vi "Global 1.vi"() -> ()   [LabVIEW 2015]
uses:
  <vilib>/Analysis/Matrix/Datatypes/RealMatrix.ctl
  <vilib>/Analysis/Matrix/NI_Matrix.lvlib
panel:
  out "LCM_CAN_EYE_RAW_T":T1={"hash"=-386282380061490012, "sys time"=0, "mobileye time"=0, "ID"=0, "data"=[]} {"hash" format="%016x"}
  out "Door":bool
  out "Right light":bool
  out "Left light":bool
  out "time":u32
  out "WHL_SPD_FL":dbl
  out "WHL_SPD_FR":dbl
  out "WHL_SPD_RL":dbl
  out "WHL_SPD_RR":dbl
  out "LCM PC":T2={"connection ID"=refnum, "net address"=0, "port"=7667}
  out "CON_INPUT_T":T3={"hash"=7122929053877479277, "sys time"=0, "ref_vel"=0.0, "ref_steer"=0.0} {"hash" format="%016x"}
  out "LCM_CON_T":T4={"hash"=4999688090526594712, "sys time"=0, "Auto"=FALSE, "Run"=FALSE, "Solenoid"=FALSE, "T lim"=FALSE, "brk_enc"=0, "B PWM"=0, "T PWM"=0, "ref_vel"=0.0, "ref_bkr_enc"=0.0, "ref_apv"=0.0, "ref_steer"=0.0} {"hash" format="%016x"}
  out "LCM_EYE_RAW_T":T5={"hash"=-8920902524919788889, "sys time"=0, "mobileye"=[]} {"hash" format="%016x"}
  out "LCM_POS_T":T6={"hash"=8611666821338907869, "sys time"=0, "dt"=0.0, "x"=0.0, "y"=0.0, "speed"=0.0, "heading"=0.0, "yaw_rate"=0.0} {"hash" format="%016x"}
  out "LCM_CAN_T":T7={"hash"=4925705798588944810, "sys time"=0, "time"=0.0, "yaw_rate"=0.0, "mdps torque"=0.0, "mdps str_ang"=0.0, "VS_CAN"=0.0, "lat_accel"=0.0, "mcp"=0.0, "accel pedal value"=0.0, "tps"=0.0, "odometer"=0.0, "battery voltage"=0.0, "WHL_SPD_RR"=0.0, "WHL_SPD_RL"=0.0, "WHL_SPD_FR"=0.0, "WHL_SPD_FL"=0.0} {"hash" format="%016x"}
  out "LCM":T2={"connection ID"=refnum, "net address"=0, "port"=7667}
  out "LCM_GGA_T":T8={"hash"=1114363806672425932, "sys time"=0, "time"=0.0, "x"=0.0, "y"=0.0, "h"=0.0, "numSV"=0, "postype"=0, "lag"=0, "hordev"=0.0, "lat"=0.0, "lon"=0.0, "hgt"=0.0, "map_idx"=0} {"hash" format="%016x"}
  out "LCM_RMC_T":T9={"hash"=2469426948741950939, "sys time"=0, "time"=0.0, "speed"=0.0, "heading"=0.0, "lat"=0.0, "lon"=0.0} {"hash" format="%016x"}
  out "K":T10=[[1.0, 0.0, 0.0], [0.0, 1.0, 0.0], [0.0, 0.0, 0.05], [0.0, 0.0, 0.0], [0.0, 0.0, 0.0]]
  out "Pp":T10=[[1.0, 0.0, 0.0, 0.0, 0.0], [0.0, 1.0, 0.0, 0.0, 0.0], [0.0, 0.0, 0.05, 0.0, 0.0], [0.0, 0.0, 0.0, 0.0188, 0.0], [0.0, 0.0, 0.0, 0.0, 0.0017]]
  out "H":T10=[[1.0, 0.0, 0.0, 0.0, 0.0], [0.0, 1.0, 0.0, 0.0, 0.0], [0.0, 0.0, 0.0, 1.0, 0.0]]
  out "R":T10=[[10.0, 0.0, 0.0], [0.0, 10.0, 0.0], [0.0, 0.0, 0.5]]
  out "Q":T10=[[0.5, 0.0, 0.0, 0.0, 0.0], [0.0, 0.5, 0.0, 0.0, 0.0], [0.0, 0.0, 0.1, 0.0, 0.0], [0.0, 0.0, 0.0, 0.0341, 0.0], [0.0, 0.0, 0.0, 0.0, 0.0017]]
  out "P":T10=[[1.0, 0.0, 0.0, 0.0, 0.0], [0.0, 1.0, 0.0, 0.0, 0.0], [0.0, 0.0, 0.1, 0.0, 0.0], [0.0, 0.0, 0.0, 0.0341, 0.0], [0.0, 0.0, 0.0, 0.0, 0.0017]]
  out "gps_pos 2":dbl[](array[numeric]) format="%#_19f"
  out "gps_vel 2":dbl[](array[numeric]) format="%#_19f"
  out "gps_pos 1":dbl[](array[numeric]) format="%#_19f"
  out "gps_vel 1":dbl[](array[numeric]) format="%#_19f"
  out "ts":dbl
  out "mcp":u16
  out "Ref Brk FULL":dbl=80.0
  out "Ref Brk Enc":dbl
  out "Ref APS":dbl
  out "VS_CAN":dbl
  out "Brake Encoder mcp":dbl
  out "mdps str_ang":dbl
  out "mdps torque":dbl
  out "vs_esc":dbl
  out "odometer":dbl
  out "gear selector disp":u8
  out "battery voltage":dbl
  out "brake_act_can":bool
  out "accel pedal value":dbl
  out "tps":dbl
  out "lat_accel":dbl
  out "yaw_rate":dbl
  out "Auto":bool
  out "Run":bool
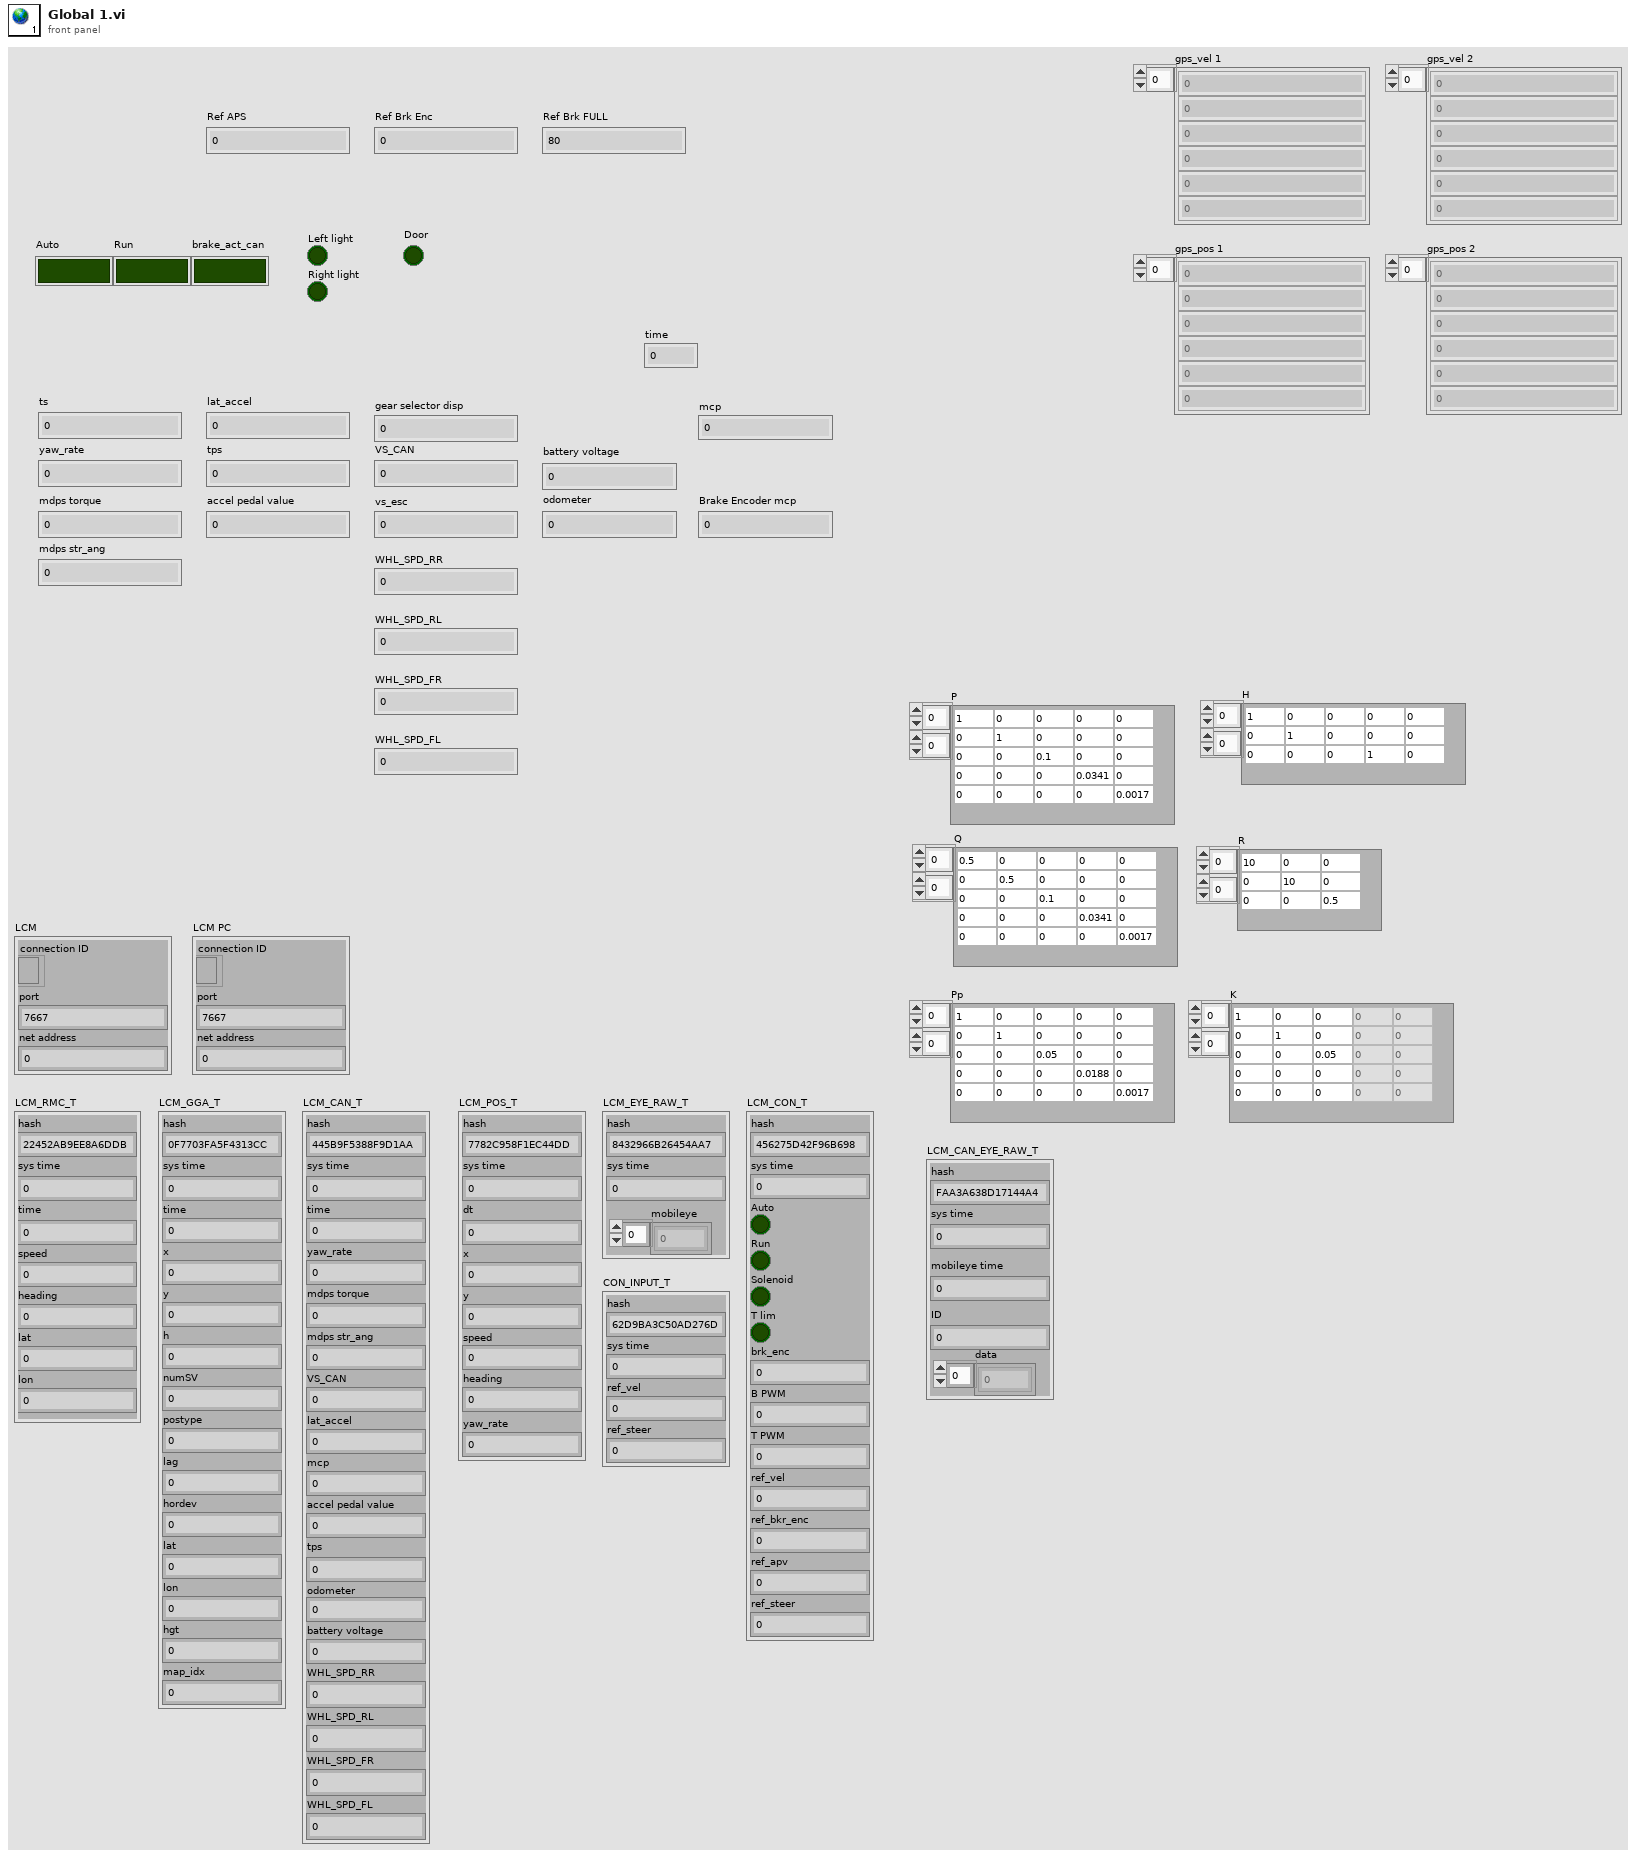
[diagram p1: front panel]
types:
  T1 = cluster{"hash":i64, "sys time":i64, "mobileye time":u32, "ID":u32, "data":u8[]}
  T2 = cluster{"connection ID":refnum<k16>, "net address":u32, "port":u16}
  T3 = cluster{"hash":i64, "sys time":i64, "ref_vel":dbl, "ref_steer":dbl}
  T4 = cluster{"hash":i64, "sys time":i64, "Auto":bool, "Run":bool, "Solenoid":bool, "T lim":bool, "brk_enc":u8, "B PWM":u16, "T PWM":u16, "ref_vel":dbl, "ref_bkr_enc":dbl, "ref_apv":dbl, "ref_steer":dbl}
  T5 = cluster{"hash":i64, "sys time":i64, "mobileye":u8[]}
  T6 = cluster{"hash":i64, "sys time":i64, "dt":dbl, "x":dbl, "y":dbl, "speed":dbl, "heading":dbl, "yaw_rate":dbl}
  T7 = cluster{"hash":i64, "sys time":i64, "time":dbl, "yaw_rate":dbl, "mdps torque":dbl, "mdps str_ang":dbl, "VS_CAN":dbl, "lat_accel":dbl, "mcp":dbl, "accel pedal value":dbl, "tps":dbl, "odometer":dbl, "battery voltage":dbl, "WHL_SPD_RR":dbl, "WHL_SPD_RL":dbl, "WHL_SPD_FR":dbl, "WHL_SPD_FL":dbl}
  T8 = cluster{"hash":i64, "sys time":i64, "time":dbl, "x":dbl, "y":dbl, "h":dbl, "numSV":i32, "postype":i32, "lag":i32, "hordev":dbl, "lat":dbl, "lon":dbl, "hgt":dbl, "map_idx":i32}
  T9 = cluster{"hash":i64, "sys time":i64, "time":dbl, "speed":dbl, "heading":dbl, "lat":dbl, "lon":dbl}
  T10 = typedef "NI_Matrix.lvlib/RealMatrix.ctl" = dbl[][]
diagram:
